vi "Save per pc label config.vi"(8 "error in (no error)":errorcluster, 9 "Darkness":string, 10 "Label right offset":string, 11 "Label down offset":string) -> (0 "error out":errorcluster)   [LabVIEW 2013]
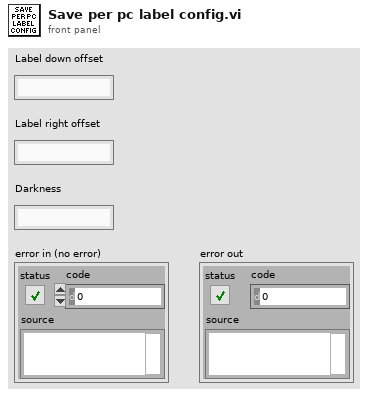
[diagram p1: front panel]
types:
  T1 = cluster{"Test folder":string, "Top level":string, "Main":string, "Test report":string, "Work order qty":string, "Work order meid":string, "Work order imei":string, "Master meid imei list":string, "Master test data":string, "ZPL label info":string, "Pictures":string, "Setup info":string, "Work order":string, "Tests folder":string, "Tests steps folder":string, "Config folder":string, "Verizon Upload file":string, "Job data file":string, "Station globals":string, "Post test info":string}
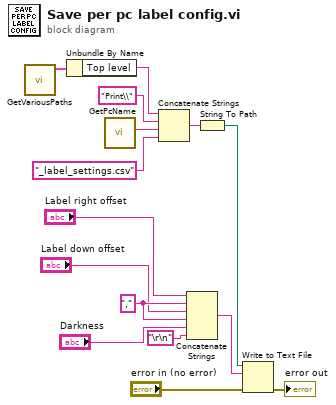
[diagram p0: block diagram]
diagram:
  w11 = "," ("string")
  n1 = call "GetVariousPaths.vi"() -> ("Built Paths"=w4:T1)  [unwired: 10 in, 1 out]
  n2 = Unbundle By Name(w4) -> ("Top level"=w3:string)
  n3 = call "GetPcName.vi"() -> ("Basic Name"=w14:string)  [unwired: 8 in, 3 out]
  n4 = Concatenate Strings(w3, "Print\\" ("string"), w14, "_label_settings.csv" ("string")) -> (w5:string)
  n5 = Concatenate Strings("Label right offset", w11, "Label down offset", w11, "Darkness", "\r\n") -> (w15:string)
  n6 = String To Path(string=w5) -> (path=w6:path)
  n7 = Write to Text File(file (use dialog)=w6, text=w15, error in="error in (no error)") -> (error out=→"error out":errorcluster)  [unwired: 1 in, 2 out]
